vi "stimulus params to string samuel.vi"(8 "error in":errorcluster, 11 "stimulus params":T1) -> (0 "error out":errorcluster, 2 "short stimulus string":string, 3 "stimulus string description":string)   [LabVIEW 2013]
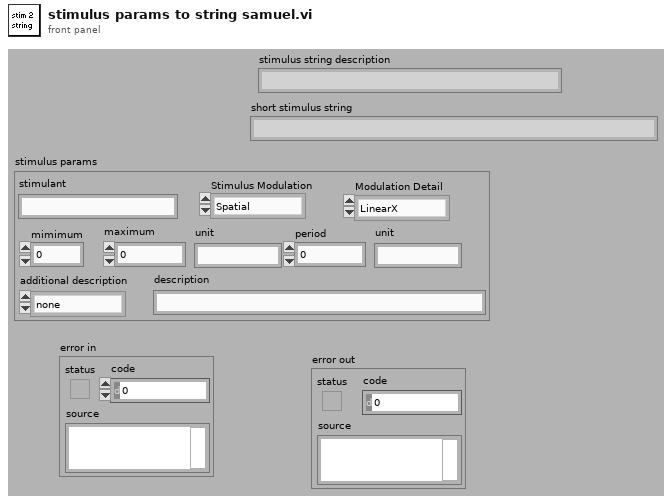
[diagram p1: front panel]
types:
  T1 = cluster{"Stimulus Modulation":enum16{"Spatial", "Temporal", "Constant", "Other"}, "stimulant":string, "maximum":u16, "mimimum":u16, "period":u16, "Modulation Detail":enum16{"LinearX", "LinearY", "Triangle", "Sine", "Square", "AngledX", "AngledY"}, "unit":string, "period_unit":string, "additional description":enum16{"none", "append", "replace"}, "description":string}
  T2 = enum16{"Spatial", "Temporal", "Constant", "Other"}
  T3 = enum16{"LinearX", "LinearY", "Triangle", "Sine", "Square", "AngledX", "AngledY"}
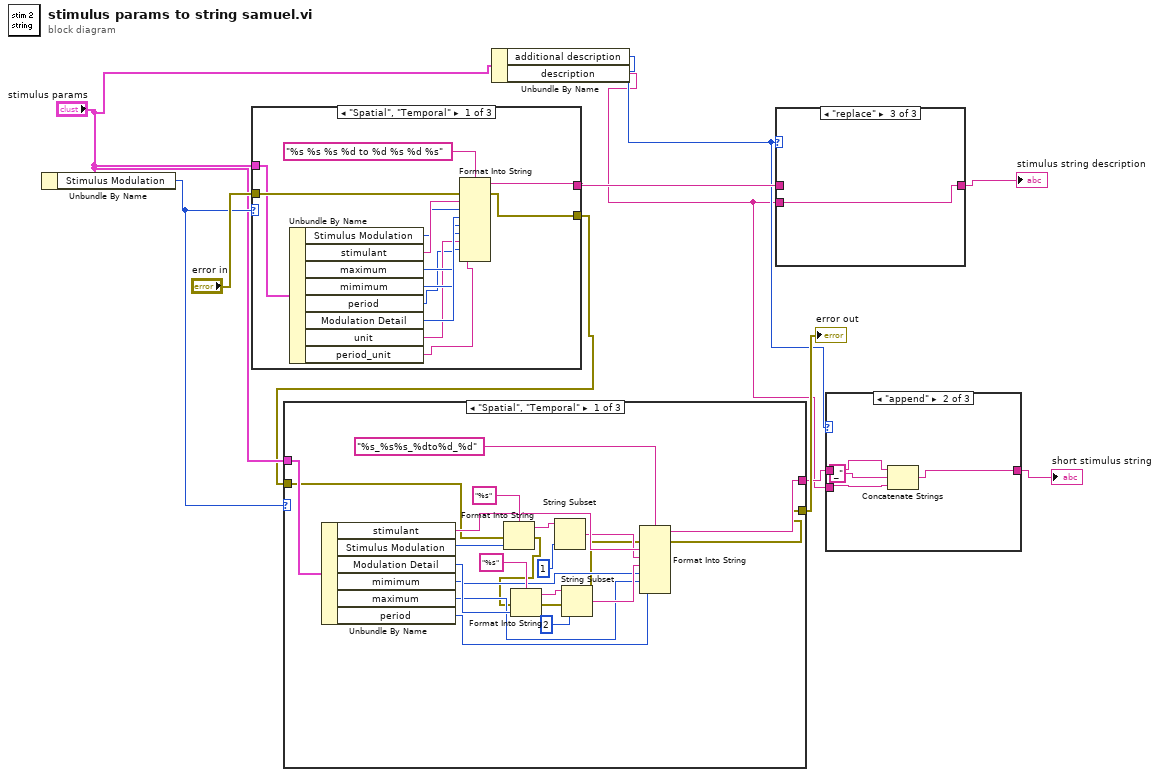
[diagram p0: block diagram]
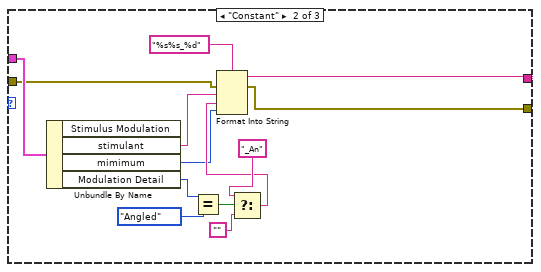
[diagram p4: hidden frame]
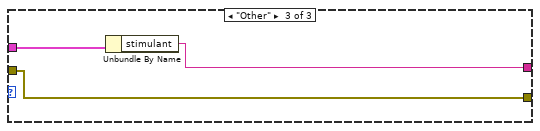
[diagram p5: hidden frame]
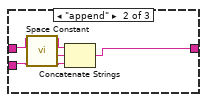
[diagram p7: hidden frame]
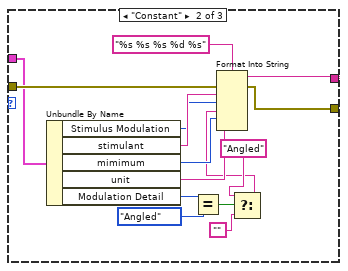
[diagram p8: hidden frame]
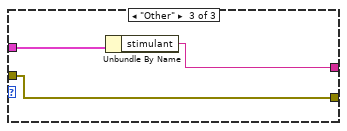
[diagram p9: hidden frame]
diagram:
  n1 = Unbundle By Name("stimulus params") -> ("Stimulus Modulation"=w8:T2)
  n2 = case shown="\"Spatial\", \"Temporal\"" w8 {
    tunnel: "error in" -> [w23 w38 w40]
    tunnel: [w22 w37 w41] -> w10
    tunnel: "stimulus params" -> [w21 w36 w42]
    tunnel: [w12 w33 w40] -> w6
    frame "Spatial", "Temporal" {
      n3 = Unbundle By Name(w21) -> ("Stimulus Modulation"=w19:T2, "stimulant"=w20:string, "maximum"=w16:u16, "mimimum"=w17:u16, "period"=w14:u16, "Modulation Detail"=w18:T3, "unit"=w15:string, "period_unit"=w13:string)
      n4 = Format Into String(format string="%s %s %s %d to %d %s %d %s", error in=w23, w20, w19, w18, w17, w16, w15, w14, w13) -> (resulting string=w22:string, error out=w12:errorcluster)  [unwired: 1 in]
    }
    frame "Constant" {
      n5 = Unbundle By Name(w36) -> ("Stimulus Modulation"=w34:T2, "stimulant"=w35:string, "mimimum"=w32:u16, "unit"=w31:string, "Modulation Detail"=w30:T3)
      n6 = Equal?(x=w30, y=enum16{"Linear", "Sine", "Square", "Angled"}."Angled") -> (x = y?=w28:bool)
      n7 = Select(t="Angled" ("unit"), s=w28, f="") -> (s? t:f=w25:string)
      n8 = Format Into String(format string="%s %s %s %d %s", error in=w38, w35, w34, w25, w32, w31) -> (resulting string=w37:string, error out=w33:errorcluster)  [unwired: 1 in]
    }
    frame "Other" {
      n9 = Unbundle By Name(w42) -> ("stimulant"=w41:string)
    }
  }
  n10 = case shown="\"Spatial\", \"Temporal\"" w8 {
    tunnel: [w47 w75 w78] -> w4
    tunnel: "stimulus params" -> [w63 w74 w79]
    tunnel: [w43 w72 w77] -> w5
    tunnel: w6 -> [w46 w64 w77]
    frame "Spatial", "Temporal" {
      n11 = Unbundle By Name(w63) -> ("stimulant"=w53:string, "Stimulus Modulation"=w61:T2, "Modulation Detail"=w56:T3, "mimimum"=w50:u16, "maximum"=w49:u16, "period"=w48:u16)
      n12 = Format Into String(format string="%s", error in=w46, w61) -> (resulting string=w60:string, error out=w45:errorcluster)  [unwired: 1 in]
      n13 = Format Into String(format string="%s", error in=w45, w56) -> (resulting string=w57:string, error out=w44:errorcluster)  [unwired: 1 in]
      n14 = String Subset(string=w60, length (rest)=1 ("length (rest)")) -> (substring=w52:string)  [unwired: 1 in]
      n15 = String Subset(string=w57, length (rest)=2 ("length (rest)")) -> (substring=w51:string)  [unwired: 1 in]
      n16 = Format Into String(format string="%s_%s%s_%dto%d_%d", error in=w44, w53, w52, w51, w50, w49, w48) -> (resulting string=w47:string, error out=w43:errorcluster)  [unwired: 1 in]
    }
    frame "Constant" {
      n17 = Unbundle By Name(w74) -> ("stimulant"=w73:string, "mimimum"=w66:u16, "Modulation Detail"=w65:T3)  [unwired: 1 out]
      n18 = Equal?(x=w65, y=enum16{"Linear", "Sine", "Square", "Angled"}."Angled") -> (x = y?=w70:bool)
      n19 = Select(t="_An" ("unit"), s=w70, f="") -> (s? t:f=w67:string)
      n20 = Format Into String(format string="%s%s_%d", error in=w64, w73, w67, w66) -> (resulting string=w75:string, error out=w72:errorcluster)  [unwired: 1 in]
    }
    frame "Other" {
      n21 = Unbundle By Name(w79) -> ("stimulant"=w78:string)
    }
  }
  "error out" <- w5
  n22 = Unbundle By Name("stimulus params") -> ("additional description"=w3:enum16{"none", "append", "replace"}, "description"=w2:string)
  n23 = case shown="\"replace\"" w3 {
    tunnel: w10 -> [w80 w83 _]
    tunnel: [w80 w81 w85] -> w9
    tunnel: w2 -> [_ w82 w85]
    frame "none", Default {
    }
    frame "append" {
      n24 = call <vilib>:"Space Constant.vi"() -> ("String"=w84:string)
      n25 = Concatenate Strings(w83, w84, w82) -> (w81:string)
    }
    frame "replace" {
    }
  }
  "stimulus string description" <- w9
  n26 = case shown="\"append\"" w3 {
    tunnel: w4 -> [w86 w90 _]
    tunnel: [w86 w88 w91] -> w1
    tunnel: w2 -> [_ w89 w91]
    frame "none", Default {
    }
    frame "append" {
      n27 = Concatenate Strings(w90, "_" ("String"), w89) -> (w88:string)
    }
    frame "replace" {
    }
  }
  "short stimulus string" <- w1
